vi "listen1.vi"() -> ()   [LabVIEW 2024]
uses:
  <vilib>/express/express analysis/Spectral/Block/exnSpectralBlock spectral measurements RMS poly.vi
  <vilib>/express/express analysis/Spectral/Block/exnSpectralBlock spectral measurements RMS array WFM.vi
  <vilib>/express/express analysis/Spectral/Block/exnSpectralBlock spectral measurements power poly.vi
  <vilib>/express/express analysis/Spectral/Block/exnSpectralBlock spectral measurements power array WFM.vi
  <vilib>/express/express analysis/Spectral/XNode/ExpressSpectralMeasurementsBlockNode.xnode
panel:
  in  "path":path
  in  "Cluster":T1={"Frequency"=500.0, "Amplitude"=1.0, "Phase"=0.0}
  in  "Simulated Inputs":T2(ring)
  out "Power Spectrum":cluster{"f0":dbl, "df":dbl, "magnitude":dbl[]}[](graph)
  out "FFT - (RMS)":cluster{"f0":dbl, "df":dbl, "magnitude":dbl[]}[](graph)
  in  "stop":bool
  out "Data":waveform(dbl)[](graph)
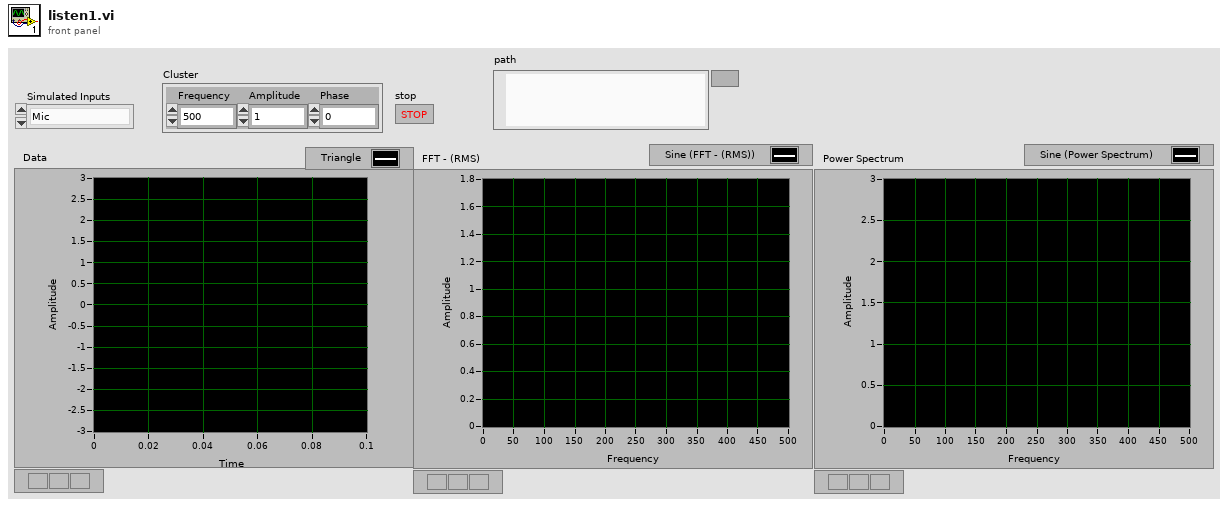
[diagram p1: front panel]
types:
  T1 = cluster{"Frequency":dbl, "Amplitude":dbl, "Phase":dbl}
  T2 = enum16{"Mic", "Sin", "Cos", "Square", "Triangle", "Files"}
  T3 = enum16{"Mic", "Sin", "Cos", "Square", "Triangle"}
  T4 = cluster{"averaging mode":u16, "weighting mode":u16, "number of averages":u32}
  T5 = cluster{"dB On (F)":bool, "unwrap phase (F)":bool, "convert to degree (F)":bool}
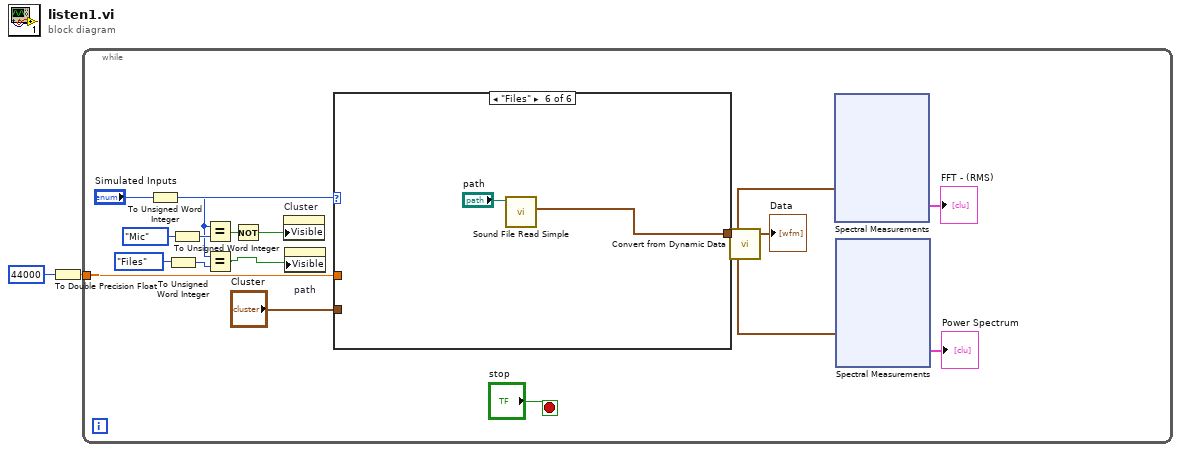
[diagram p0: block diagram]
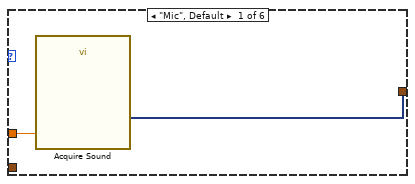
[diagram p2: hidden frame]
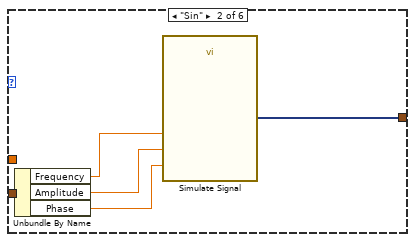
[diagram p3: hidden frame]
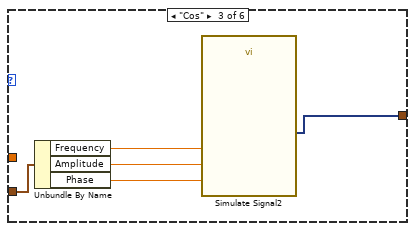
[diagram p4: hidden frame]
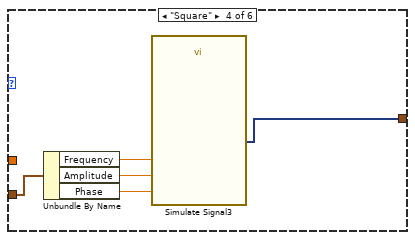
[diagram p5: hidden frame]
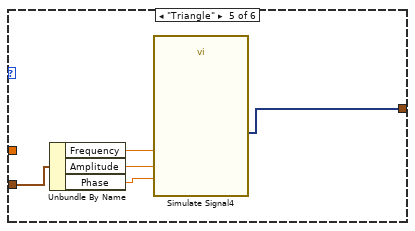
[diagram p6: hidden frame]
diagram:
  n1 = To Double Precision Float(number=44000) -> (double precision float=w1:dbl)
  n2 = while {
    tunnel: w1 -> [w14]
    stop <- "stop" stop-if-true
    n3 = To Unsigned Word Integer(number="Simulated Inputs") -> (unsigned 16bit integer=w5:u16)
    n4 = To Unsigned Word Integer(number=T2."Files" ("Simulated Inputs")) -> (unsigned 16bit integer=w4:u16)
    n5 = To Unsigned Word Integer(number=T3."Mic" ("y")) -> (unsigned 16bit integer=w7:u16)
    n6 = Equal?(x=w5, y=w7) -> (x = y?=w9:bool)
    n7 = Equal?(x=w5, y=w4) -> (x = y?=w3:bool)
    n8 = Not(x=w9) -> (.not. x?=w8:bool)
    n9 = property on="Cluster" class="Clust (strict)"("Visible"=w8) -> ()  [unwired: 2 in, 2 out]
    n10 = property on="path" class="Path"("Visible"=w3) -> ()  [unwired: 2 in, 2 out]
    n11 = case shown="\"Files\"" "Simulated Inputs" {
      tunnel: w14 -> [w20 _ _ _ _ _]
      tunnel: [w19 w25 w29 w31 w36 w41] -> w13
      tunnel: "Cluster" -> [_ w24 w30 w35 w40 _]
      frame "Mic", Default {
        n12 = call "Acquire Sound"("Sample rate (Hz)"=w20) -> ("Data"=w19:dynamicdata)  [unwired: 17 in, 1 out]
      }
      frame "Sin" {
        n13 = Unbundle By Name(w24) -> ("Frequency"=w23:dbl, "Amplitude"=w22:dbl, "Phase"=w21:dbl)
        n14 = call "Simulate Signal"("Frequency"=w23, "Amplitude"=w22, "Phase"=w21) -> ("Sine"=w25:dynamicdata)  [unwired: 11 in, 1 out]
      }
      frame "Cos" {
        n15 = Unbundle By Name(w30) -> ("Frequency"=w28:dbl, "Amplitude"=w27:dbl, "Phase"=w26:dbl)
        n16 = call "Simulate Signal2"("Frequency"=w28, "Amplitude"=w27, "Phase"=w26) -> ("Sine"=w29:dynamicdata)  [unwired: 11 in, 1 out]
      }
      frame "Square" {
        n17 = Unbundle By Name(w35) -> ("Frequency"=w34:dbl, "Amplitude"=w33:dbl, "Phase"=w32:dbl)
        n18 = call "Simulate Signal3"("Frequency"=w32, "Amplitude"=w33, "Phase"=w34) -> ("Square"=w31:dynamicdata)  [unwired: 11 in, 1 out]
      }
      frame "Triangle" {
        n19 = Unbundle By Name(w40) -> ("Frequency"=w39:dbl, "Amplitude"=w38:dbl, "Phase"=w37:dbl)
        n20 = call "Simulate Signal4"("Frequency"=w39, "Amplitude"=w38, "Phase"=w37) -> ("Triangle"=w36:dynamicdata)  [unwired: 11 in, 1 out]
      }
      frame "Files" {
        n21 = call <vilib>:"Sound File Read Simple.vi"("path"="path") -> ("data"=w41:waveform(dbl)[])  [unwired: 7 in, 3 out]
      }
    }
    n22 = call "Convert from Dynamic Data"("Dynamic Data Type"=w13) -> ("Array of Waveform"=→"Data":waveform(dbl)[])  [unwired: 3 in]
    n23 = xnode "Spectral Measurements"("Signals"=w13) -> ("FFT - (RMS)"=→"FFT - (RMS)":cluster{"f0":dbl, "df":dbl, "magnitude":dbl[]}[])  [unwired: 1 in, 2 out]
    n24 = xnode "Spectral Measurements"("Signals"=w13) -> ("Power Spectrum"=→"Power Spectrum":cluster{"f0":dbl, "df":dbl, "magnitude":dbl[]}[])  [unwired: 1 in, 1 out]
  }
